vi "Tulip handler Tester.vi"() -> ()   [LabVIEW 2021]
panel:
  out "Status String 2":string
  out "Response body 2":string
  out "Status String":string
  out "Response body":string
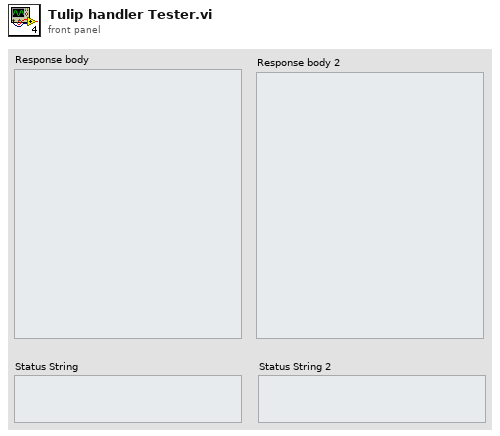
[diagram p1: front panel]
types:
  T1 = cluster{"hlscw_parametro":string, "id":string, "ntooc_date":string, "vthmf_serial_number":string, "zgnrg_result":string}
  T2 = enum16{"Init", "Get headers", "Get", "Post", "Put", "Close"}
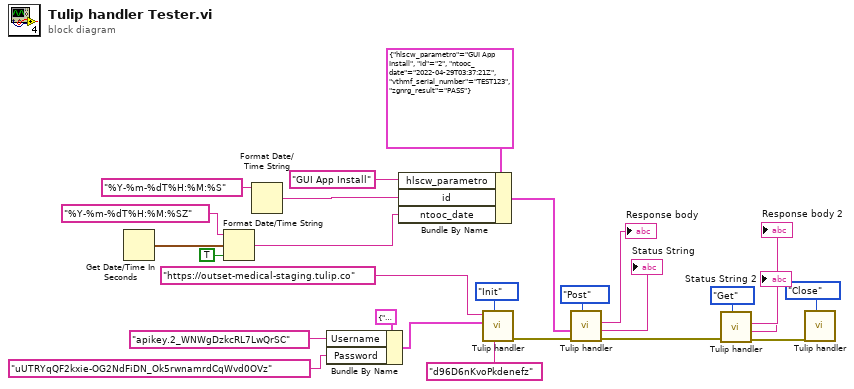
[diagram p0: block diagram]
diagram:
  n1 = Get Date/Time In Seconds() -> (seconds since 1Jan1904=w3:timestamp)
  n2 = Format Date/Time String(time format string (%c)="%Y-%m-%dT%H:%M:%SZ", seconds (now)=w3, UTC format=TRUE) -> (date/time string=w1:string)
  n3 = Format Date/Time String(time format string (%c)="%Y-%m-%dT%H:%M:%S") -> (date/time string=w7:string)  [unwired: 2 in]
  n4 = Bundle By Name(cluster=cluster{"Username":string, "Password":string} {"Username"="apikey.2_WNWgDzkcRL7LwQrSC", "Password"="uUTRYqQF2kxie-OG2NdFiDN_Ok5rwnamrdCqWvd0OVz"} ("Authentication"), "Username"="apikey.2_WNWgDzkcRL7LwQrSC", "Password"="uUTRYqQF2kxie-OG2NdFiDN_Ok5rwnamrdCqWvd0OVz") -> (w23:cluster{"Username":string, "Password":string})
  n5 = Bundle By Name(cluster=T1 {"hlscw_parametro"="GUI App Install", "id"="2", "ntooc_date"="2022-04-29T03:37:21Z", "vthmf_serial_number"="TEST123", "zgnrg_result"="PASS"} ("body"), "hlscw_parametro"="GUI App Install", "id"=w7, "ntooc_date"=w1) -> (w5:T1)
  n6 = call "Tulip handler.vi"("Table ID"="d96D6nKvoPkdenefz", "State"=T2."Init", "Authentication"=w23, "URL"="https://outset-medical-staging.tulip.co") -> ("error out"=w26:errorcluster)  [unwired: 5 in, 2 out]
  n7 = call "Tulip handler.vi"("State"=T2."Post", "error in"=w26, "Body"=w5) -> ("error out"=w17:errorcluster, "Status String"=→"Status String":string, "Response body"=→"Response body":string)  [unwired: 6 in]
  n8 = call "Tulip handler.vi"("State"=T2."Get", "error in"=w17) -> ("error out"=w15:errorcluster, "Status String"=→"Status String 2":string, "Response body"=→"Response body 2":string)  [unwired: 7 in]
  n9 = call "Tulip handler.vi"("State"=T2."Close", "error in"=w15) -> ()  [unwired: 7 in, 3 out]
